vi "Create.vi"(8 "error in (no error)":errorcluster, 10 "Channel":u8, 11 "ILC ADC Factory in":refnum<class "ILC ADC Factory.lvclass">) -> (0 "error out":errorcluster, 2 "ILC ADC":refnum<class "ILC ADC.lvclass">, 3 "ILC ADC Factory out":refnum<class "ILC ADC Factory.lvclass">)   [LabVIEW 2015, in "ILC ADC Factory.lvclass"]
uses:
  ILC ADC Factory.lvclass
  ILC ADC/ILC ADC.lvclass
  ILC ADC 1/ILC ADC 1.lvclass
  ILC ADC 2/ILC ADC 2.lvclass
  ILC ADC 3/ILC ADC 3.lvclass
  ILC ADC 4/ILC ADC 4.lvclass
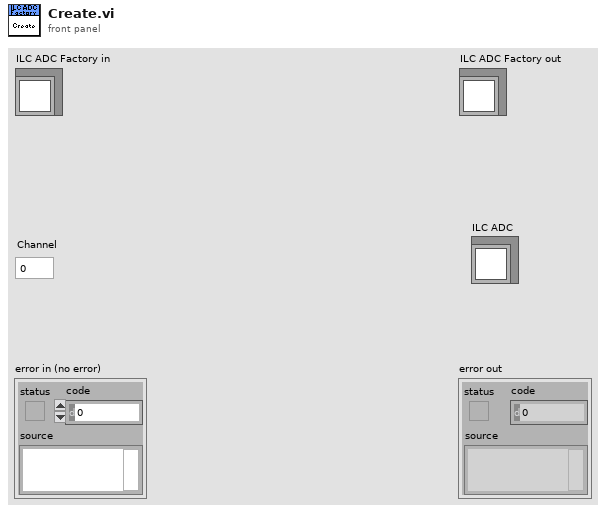
[diagram p1: front panel]
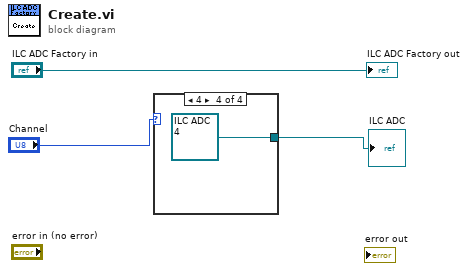
[diagram p0: block diagram]
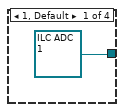
[diagram p2: hidden frame]
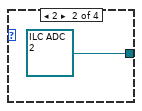
[diagram p3: hidden frame]
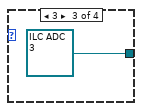
[diagram p4: hidden frame]
diagram:
  n1 = case shown="4" "Channel" {
    tunnel: [refnum<class "ILC ADC 1.lvclass"> refnum ("ILCADC1.lvclass") refnum<class "ILC ADC 2.lvclass"> refnum ("ILCADC2.lvclass") refnum<class "ILC ADC 3.lvclass"> refnum ("ILCADC3.lvclass") refnum<class "ILC ADC 4.lvclass"> refnum ("ILCADC4.lvclass")] -> w1
    frame 1, Default {
    }
    frame 2 {
    }
    frame 3 {
    }
    frame 4 {
    }
  }
  "ILC ADC" <- w1
  "ILC ADC Factory out" <- "ILC ADC Factory in"
